vi "NATS Stop Monitor.vi"(8 "error in":errorcluster, 11 "async monitor":refnum<vi>) -> (0 "error out":errorcluster)   [LabVIEW 2023, in "NATS Core.lvlib"]
doc: "Reads a message from the NATS server."
uses:
  NATS Core.lvlib
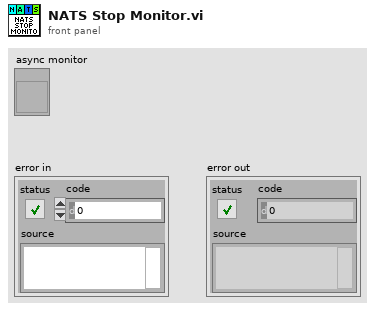
[diagram p1: front panel]
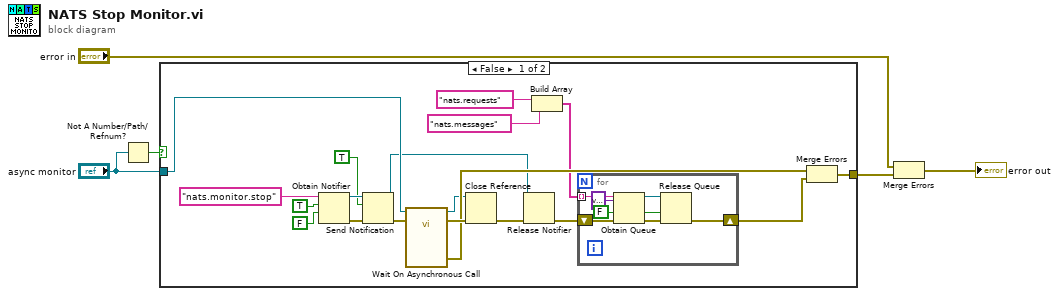
[diagram p0: block diagram]
diagram:
  n1 = Not A Number/Path/Refnum?(number/path/refnum="async monitor") -> (NaN/Path/Refnum?=w1:bool)
  n2 = case shown="False" w1 {
    tunnel: [w21 _] -> w5
    tunnel: "async monitor" -> [w13 _]
    frame False {
      n3 = Obtain Notifier(name (unnamed)="nats.monitor.stop", notification data type=TRUE, create if not found? (T)=FALSE) -> (notifier out=w16:refnum<notifier>, error out=w23:errorcluster)  [unwired: 1 in, 1 out]
      n4 = Send Notification(notification=TRUE, notifier=w16, error in (no error)=w23) -> (notifier out=w12:refnum<notifier>, error out=w22:errorcluster)
      n5 = call-by-ref "Wait On Asynchronous Call"(reference=w13, error in=w22) -> (reference out=w14:refnum<vi>, error out=w24:errorcluster, 0:"error out"=w20:errorcluster)  [unwired: 11 in]
      n6 = Close Reference(reference=w14, error in (no error)=w24) -> (error out=w11:errorcluster)
      n7 = Release Notifier(notifier=w12, error in (no error)=w11) -> (error out=w10:errorcluster)  [unwired: 1 in, 2 out]
      n8 = Build Array("nats.requests" ("name (unnamed)"), "nats.messages" ("name (unnamed)")) -> (w6:string[])
      n9 = for {
        shift-right: [w32] -> w9
        shift-left: w10 -> [w29]
        tunnel: w6 -> [w27] mode=indexing
        n10 = Obtain Queue(name (unnamed)=w27, element data type=variant, create if not found? (T)=FALSE, error in (no error)=w29) -> (queue out=w31:refnum<queue>, created new?=w30:bool, error out=w28:errorcluster)  [unwired: 1 in]
        n11 = Release Queue(queue=w31, force destroy? (F)=w30, error in (no error)=w28) -> (error out=w32:errorcluster)  [unwired: 2 out]
      }
      n12 = Merge Errors(w20, w9) -> (w21:errorcluster)
    }
    frame True {
    }
  }
  n13 = Merge Errors("error in", w5) -> (→"error out":errorcluster)
